vi "ASK 2bits.vi"() -> ()   [LabVIEW 2010]
panel:
  out "Tableau 2":bool[](array[boolean])
  out "Graphe déroulant":dynamicdata(graph)
  in  "Tableau":bool[](array[boolean])
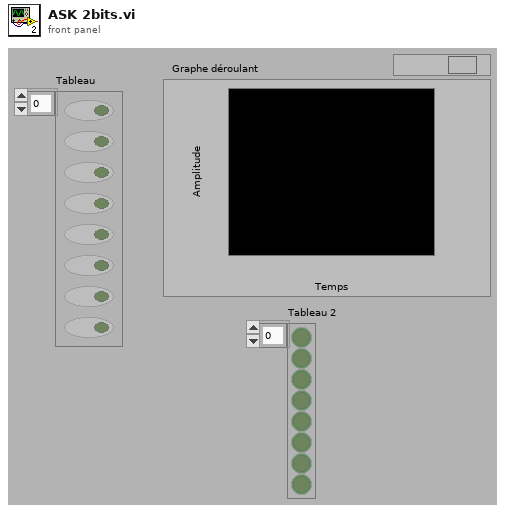
[diagram p1: front panel]
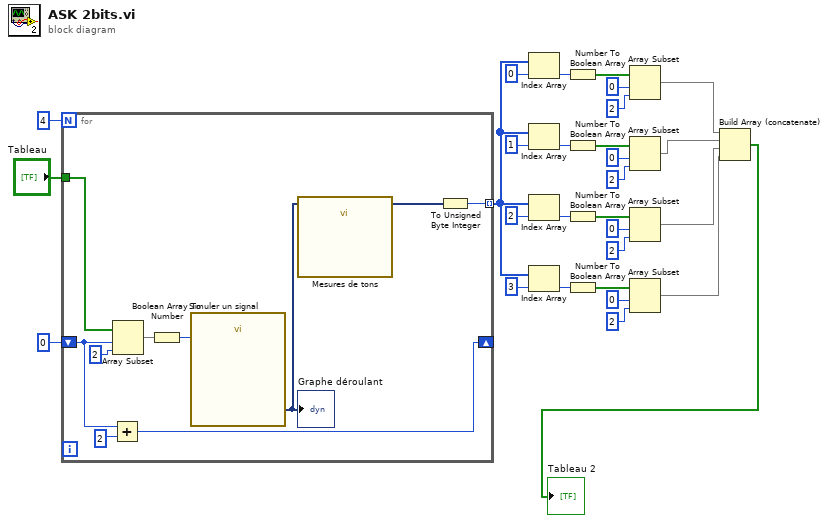
[diagram p0: block diagram]
diagram:
  n1 = for {
    N: 4 -> [_]
    shift-right: [w38] -> _
    shift-left: 0 -> [w37]
    tunnel: "Tableau" -> [w35]
    tunnel: [w30] -> w22 mode=indexing
    n2 = Add(x=w37, y=2) -> (x+y=w38:i32)
    n3 = Array Subset(array=w35, index=w37, length=2) -> (w34:bool[])
    n4 = Boolean Array To Number(Boolean array=w34) -> (number=w33:u32)
    n5 = call "Simuler un signal"("Amplitude"=w33) -> ("Sinus"=w32:dynamicdata)  [unwired: 13 in, 1 out]
    "Graphe déroulant" <- w32
    n6 = call "Mesures de tons"("Signals"=w32) -> ("Amplitude"=w31:dynamicdata)  [unwired: 7 in, 3 out]
    n7 = To Unsigned Byte Integer(number=w31) -> (unsigned 8bit integer=w30:u8)
  }
  n8 = Index Array(array=w22, index=0) -> (element=w7:u8)
  n9 = Index Array(array=w22, index=1) -> (element=w9:u8)
  n10 = Index Array(array=w22, index=2) -> (element=w12:u8)
  n11 = Index Array(array=w22, index=3) -> (element=w13:u8)
  n12 = Number To Boolean Array(number=w7) -> (Boolean array=w6:bool[])
  n13 = Number To Boolean Array(number=w9) -> (Boolean array=w8:bool[])
  n14 = Number To Boolean Array(number=w12) -> (Boolean array=w11:bool[])
  n15 = Number To Boolean Array(number=w13) -> (Boolean array=w10:bool[])
  n16 = Array Subset(array=w6, index=0, length=2) -> (w5:bool[])
  n17 = Array Subset(array=w8, index=0, length=2) -> (w4:bool[])
  n18 = Array Subset(array=w11, index=0, length=2) -> (w3:bool[])
  n19 = Array Subset(array=w10, index=0, length=2) -> (w2:bool[])
  n20 = Build Array (concatenate)(w5, w4, w3, w2) -> (→"Tableau 2":bool[])
